vi "saveJobData.vi"(7 "Job data xml":string, 8 "error in (no error)":errorcluster, 9 "File name wo extension":string="Test", 10 "Storage location":u16(ring)=1 items=["Flash"=1, "USB"=2], 11 "SM1000-control in":T1) -> (0 "error out":errorcluster, 3 "SM1000-control out":T1)   [LabVIEW 2013, in "SLMControl.lvlib" / "SM1000.lvclass"]
doc: "Send job data for storage in the EC1000 flash memory or USB device.\n\nJob data is compiled and stored on the target EC1000 Flash file system for use in Local Mode."
uses:
  SM1000.lvclass
  Object-reference.ctl
  SM1000.lvclass/SM1000.ctl
  Custom-errors.ctl
  C:/Users/vangeste/Desktop/2015-06-02 - SLM - MAIF/HC-HardwareCharacterization/Sources/SM1000/LECSession.dll
  HC-HardwareCharacterization/Sources/SM1000/LECSession.dll
  DOTNET-error-int.vi
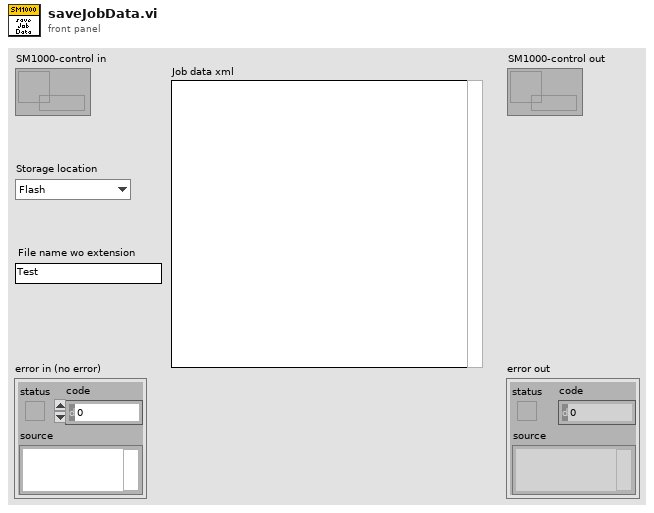
[diagram p1: front panel]
types:
  T1 = typedef "SLMControl.lvlib/SM1000.lvclass/Object-reference.ctl" = refnum<data-value>
  T2 = typedef "SLMControl.lvlib/SM1000.lvclass/Custom-errors.ctl" = enum16{"No error", "Not implemented", "Command not recognized", "Invalid input", "No connection", "Timeout", "Resource not loaded"}
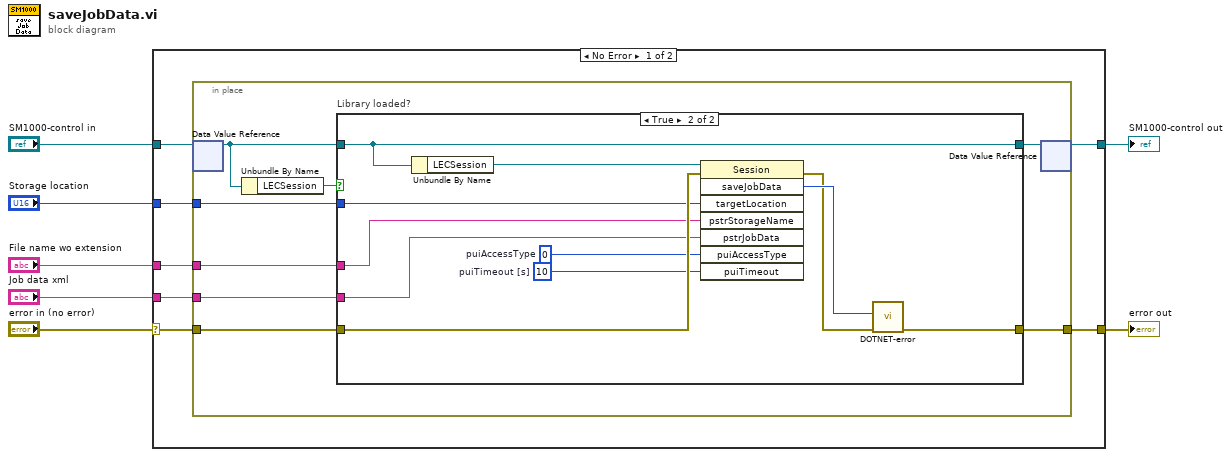
[diagram p0: block diagram]
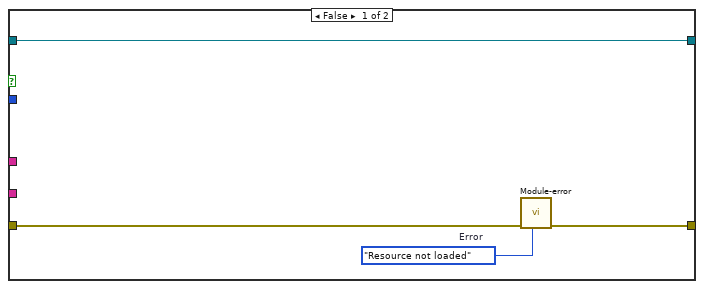
[diagram p2: hidden frame]
diagram:
  n1 = case shown="No Error" "error in (no error)" {
    selector: "error in (no error)" -> [w12 w39]
    tunnel: [w11 w39] -> w6
    tunnel: [w13 w38] -> w4
    tunnel: "SM1000-control in" -> [w14 w38]
    tunnel: "File name wo extension" -> [w10 _]
    tunnel: "Job data xml" -> [w9 _]
    tunnel: "Storage location" -> [w8 _]
    frame No Error {
      n2 = in-place {
        in-place-border: w12 -> [w22]
        in-place-border: [w19] -> w11
        in-place-border: w10 -> [w17]
        in-place-border: w9 -> [w16]
        in-place-border: w8 -> [w15]
        n3 = in-place-dvr #1(w14) -> (w20:refnum<class "SM1000.lvclass">)  [unwired: 1 out]
        n4 = Unbundle By Name(w20) -> ("LECSession"=w21:bool)
        n5 = case "Library loaded?" shown="True" w21 {
          tunnel: w22 -> [w26 w36]
          tunnel: w20 -> [w24 w34]
          tunnel: [w25 w29] -> w19
          tunnel: [w24 w34] -> w18
          tunnel: w17 -> [_ w35]
          tunnel: w16 -> [_ w30]
          tunnel: w15 -> [_ w33]
          frame False {
            w23 = Custom-errors."Resource not loaded"  # Error
            n6 = call "Module-error.vi"("Error"=w23, "error in (no error)"=w26) -> ("error out"=w25:errorcluster)  [unwired: 9 in]
          }
          frame True {
            w31 = u32 0  # puiAccessType
            w32 = u32 10  # puiTimeout [s]
            n7 = Unbundle By Name(w34) -> ("LECSession"=w37:refnum<k24>)
            n8 = invoke class="Session" method="saveJobData"(reference=w37, error in=w36, "targetLocation"=w33, "pstrStorageName"=w35, "pstrJobData"=w30, "puiAccessType"=w31, "puiTimeout"=w32) -> (error out=w27:errorcluster, "saveJobData"=w28:u32)  [unwired: 1 in, 6 out]
            n9 = call-poly "DOTNET-error.vi"("error in (no error)"=w27, "Retun code"=w28) -> ("error out"=w29:errorcluster)  [unwired: 9 in]
          }
        }
        n10 = in-place-dvr #1(w18) -> (w13:T1)  [unwired: 1 out]
      }
    }
    frame Error {
    }
  }
  "error out" <- w6
  "SM1000-control out" <- w4
